vi "Client (SubVI).vi"(11 "String":string) -> ()   [LabVIEW 2023]
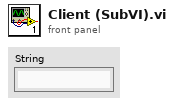
[diagram p1: front panel]
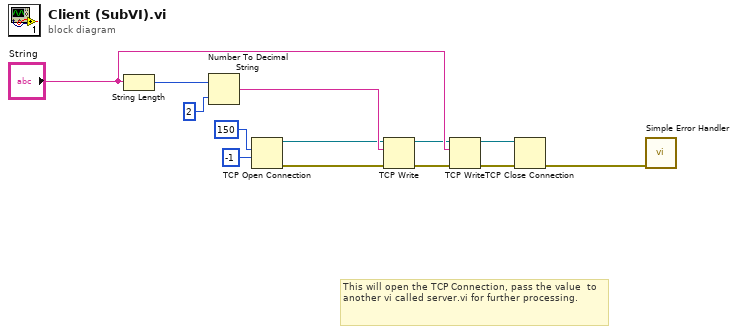
[diagram p0: block diagram]
diagram:
  # "This will open the TCP Connection, pass the value  to another vi called server.vi for further processing."
  n1 = String Length(string="String") -> (length=w10:i32)
  n2 = Number To Decimal String(number=w10, width (-)=2) -> (decimal integer string=w13:string)
  n3 = TCP Open Connection(remote port or service name=u16 150, timeout ms (60000)=-1) -> (connection ID=w6:refnum<k5>, error out=w8:errorcluster)  [unwired: 3 in]
  n4 = TCP Write(connection ID=w6, data in=w13, error in (no error)=w8) -> (connection ID out=w7:refnum<k5>, error out=w9:errorcluster)  [unwired: 1 in, 1 out]
  n5 = TCP Write(connection ID=w7, data in="String", error in (no error)=w9) -> (connection ID out=w3:refnum<k5>, error out=w2:errorcluster)  [unwired: 1 in, 1 out]
  n6 = TCP Close Connection(connection ID=w3, error in (no error)=w2) -> (error out=w1:errorcluster)  [unwired: 1 in, 1 out]
  n7 = call <vilib>:"Simple Error Handler.vi"("error in (no error)"=w1) -> ()  [unwired: 4 in, 5 out]
